vi "HLA Custom Device.Async.vi"(10 "Parameters":variant, 11 "Process":refnum<class "Process.lvclass">) -> ()   [LabVIEW 2019, in "HLA Custom Device Engine.lvlib"]
uses:
  HLA Custom Device Engine.lvlib
  <vilib>/NI/NIVS Inline Async API/_VS Inline Async API/Process/Process.lvclass
  _typedefs/AsyncDataSpace.ctl
  <vilib>/NI/NIVS Inline Async API/_Data Access Engine/Data Access Engine/Types/Write.DVR.ctl
  <vilib>/NI/NIVS Inline Async API/_Data Access Engine/Access Type Classes/Write/Write.lvclass
  <vilib>/NI/NIVS Inline Async API/_VS Inline Async API/Process/Process.lvclass/Process.ctl
  RTruntimeData.ctl
  _typedefs/RThlaMapHelpers.ctl
  _typedefs/map_in_interaction.ctl
  _typedefs/map_interaction_value.ctl
  _typedefs/map_attr_param_data.ctl
  _typedefs/map_object.ctl
  _typedefs/map_object_key.ctl
  _typedefs/map_object_value.ctl
  _typedefs/map_object_instance.ctl
  _typedefs/map_object_instance_value.ctl
  _typedefs/map_object_vs_instance.ctl
  _typedefs/map_out_vs_ch_instanceId.ctl
  _typedefs/map_out_vs_ch_objects.ctl
  _typedefs/map_out_vs_ch_objects_value.ctl
  _typedefs/map_out_vs_ch_interactIonClass.ctl
  <vilib>/addons/hla/receiveInteractionEvent_type.ctl
  <vilib>/addons/hla/OrderType.ctl
  <vilib>/addons/hla/TransportationType.ctl
  <vilib>/addons/hla/reflectAttributeValuesEvent_type.ctl
  <vilib>/addons/hla/discoverObjectInstanceEvent_type.ctl
  <vilib>/addons/hla/removeObjectInstanceEvent_type.ctl
  <vilib>/NI VeriStand/Custom Device API/Block Data Reference.ctl
  <vilib>/NI VeriStand/Custom Device API/Data Reference.ctl
  _typedefs/receiveInteraction_type.ctl
  _typedefs/interaction_info_incoming_type.ctl
  _typedefs/dataElement_type.ctl
  _typedefs/reflectAttributeValues_type.ctl
  _typedefs/object_info_received_type.ctl
  _typedefs/discoverObjectInstance_type.ctl
  <vilib>/NI/NIVS Inline Async API/_Data Access Engine/Access Type Classes/Write/Write.lvclass/Write.ctl
  <vilib>/NI/NIVS Inline Async API/_Data Access Engine/Data Access Engine/Methods/Write.Data.vi
  <vilib>/NI/NIVS Inline Async API/_VS Inline Async API/Process/Data Member Access/Read Data Access.vi
  <vilib>/NI/NIVS Inline Async API/_VS Inline Async API/Error Handling Process/SubVIs/Error.ConvertArray.vi
  <vilib>/NI/NIVS Inline Async API/_Data Access Engine/Access Type Classes/Write/Write.ProcessData.vi
  <vilib>/NI/NIVS Inline Async API/_Data Access Engine/Access Type Classes/Write/Write.Buffer.vi
  <vilib>/NI/NIVS Inline Async API/_Data Access Engine/Access Type Classes/Write/Write.Commit.vi
  Shared/Constants.vi
  <vilib>/NI/NIVS Inline Async API/_Data Access Engine/Data Access Engine/Methods/Write.Lookup.vi
  _subVIs/MessageQueue/Enqueue Message (Single).vi
  <vilib>/NI/NIVS Inline Async API/_Data Access Engine/Data Access Engine/Data Access Engine.lvclass
  Shared/HLA Custom Device Shared.lvlib
  _subVIs/MessageQueue/Message Queue.lvlib
  _subVIs/UserEvents/User Events.lvlib
  Shared/main_page_config.ctl
  Shared/object_attribute_configuration.ctl
  Shared/interaction_parameter_configuration.ctl
  Shared/Compiled.Settings.ctl
  <vilib>/addons/hla/helpers/ahvm.lvlib
  <vilib>/addons/hla/helpers/phvm.lvlib
  <vilib>/addons/hla/openrti_rti1516eLv.lvlib
  <vilib>/NI VeriStand/Custom Device API/Custom Device API.lvlib
  Shared/object_data.ctl
  Shared/object_status_info.ctl
  Shared/object_managament_config.ctl
  _Debug/VsDebugLibrary.lvlib
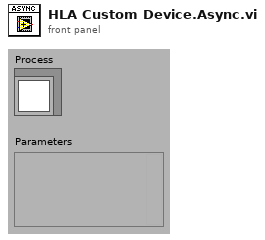
[diagram p1: front panel]
types:
  T1 = typedef "HLA Custom Device Engine.lvlib/AsyncDataSpace.ctl" = cluster{"interaction in":T2, "interaction in values":dbl[], "object in":T2, "object in values":dbl[], "status":T2, "status values":dbl[]}
  T2 = typedef "Data Access Engine.lvlib/Data Access Engine.lvclass/Write.DVR.ctl" = refnum<data-value>
  T3 = typedef "HLA Custom Device Shared.lvlib/Compiled.Settings.ctl" = cluster{"Name":string, "Async Init Timeout":u16, "main page properties":T4, "obiectConfig":T5, "objectStatus":T8, "objectData":T9}
  T4 = typedef "HLA Custom Device Shared.lvlib/main_page_config.ctl" = cluster{"Federate Execution Name":string, "Federate Type":string, "Local Designator Settings":string, "FOM Module":path, "mak mtl file":path, "FOM destination path":string, "MTL destination path":string}
  T5 = typedef "HLA Custom Device Shared.lvlib/object_managament_config.ctl" = cluster{"incoming interactions":T6[], "incoming objects":T7[], "outgoing interactions":T6[], "outgoing objects":T7[]}
  T6 = typedef "HLA Custom Device Shared.lvlib/interaction_parameter_configuration.ctl" = cluster{"interaction class name":string, "parameter name":string, "datatype":string, "vsChIndex":i32, "vsObjectId":string}
  T7 = typedef "HLA Custom Device Shared.lvlib/object_attribute_configuration.ctl" = cluster{"object class name":string, "instanceId":i32, "attribute name":string, "datatype":string, "vsChIndex":i32, "vsObjectId":string}
  T8 = typedef "HLA Custom Device Shared.lvlib/object_status_info.ctl" = cluster{"incoming interactions":map{string, map{string, i32}}, "incoming objects":map{string, map{string, i32}}, "outgoing interactions":map{string, map{string, i32}}, "outgoing objects":map{string, map{string, i32}}}
  T9 = typedef "HLA Custom Device Shared.lvlib/object_data.ctl" = cluster{"out interaction data BD":T10[], "out interaction data size":i32, "out interaction status BD":T10[], "out interaction status size":i32, "out object data BD":T10[], "out object data size":i32, "out object status BD":T10[], "out object status size":i32}
  T10 = typedef "Custom Device API.lvlib/Block Data Reference.ctl" = cluster{"Data Reference":T11, "Offset":u64, "Length":u64}
  T11 = typedef "Custom Device API.lvlib/Data Reference.ctl" = i32
  T12 = typedef "HLA Custom Device Engine.lvlib/RTruntimeData.ctl" = cluster{"rtiHandle":i64, "hlaMap":T13, "hla event registration":refnum<event-registration>, "out interaction data BD":T10[], "out interaction data":dbl[], "out interaction status BD":T10[], "out interaction status ":dbl[], "out object data BD":T10[], "out object data":dbl[], "out object status BD":T10[], "out object status ":dbl[]}
  T13 = typedef "HLA Custom Device Engine.lvlib/RThlaMapHelpers.ctl" = cluster{"in_interactionMap":T14, "in_objectMap":T17, "in_map_object_instance":T20, "in_map_vs_incoming_instance":T22, "out_map_vs_ch_instanceId":T23, "out_interactionMap":T14, "out_map_vs_ch_objectInstance":T24, "out_objectMap":T17, "out_map_vs_ch_interactionClass":T26}
  T14 = typedef "HLA Custom Device Engine.lvlib/map_in_interaction.ctl" = map{u64, T15}
  T15 = typedef "HLA Custom Device Engine.lvlib/map_interaction_value.ctl" = cluster{"infoChMap":map{string, i32}, "parameterMap":map{u64, T16}, "parHandleValueMap":u64}
  T16 = typedef "HLA Custom Device Engine.lvlib/map_attr_param_data.ctl" = cluster{"dataType":string, "offset":i32, "numOfElements":i32}
  T17 = typedef "HLA Custom Device Engine.lvlib/map_object.ctl" = map{T18, T19}
  T18 = typedef "HLA Custom Device Engine.lvlib/map_object_key.ctl" = cluster{"instanceId":i32, "objectClassHandle":u64}
  T19 = typedef "HLA Custom Device Engine.lvlib/map_object_value.ctl" = cluster{"infoChMap":map{string, i32}, "attributeMap":map{u64, T16}, "attrHandleSet":u64, "attrHandleValueMap":u64, "objectInstancePrefix":string}
  T20 = typedef "HLA Custom Device Engine.lvlib/map_object_instance.ctl" = map{u64, T21}
  T21 = typedef "HLA Custom Device Engine.lvlib/map_object_instance_value.ctl" = cluster{"objectClassHandle":u64, "objectInstanceName":string, "InstanceID":i32}
  T22 = typedef "HLA Custom Device Engine.lvlib/map_object_vs_instance.ctl" = map{u64, map{i32, u64}}
  T23 = typedef "HLA Custom Device Engine.lvlib/map_out_vs_ch_instanceId.ctl" = map{i32, i32}
  T24 = typedef "HLA Custom Device Engine.lvlib/map_out_vs_ch_objects.ctl" = map{i32, T25}
  T25 = typedef "HLA Custom Device Engine.lvlib/map_out_vs_ch_objects_value.ctl" = cluster{"objectInstanceHandle":u64, "objectClassHandle":u64}
  T26 = typedef "HLA Custom Device Engine.lvlib/map_out_vs_ch_interactIonClass.ctl" = map{i32, u64}
  T27 = typedef "HLA Custom Device Engine.lvlib/Message Queue.lvlib/All Message Queues.ctl" = cluster{"UI":refnum<queue>}
  T28 = typedef "HLA Custom Device Engine.lvlib/User Events.lvlib/userEvents_type.ctl" = cluster{"events":cluster{"stop":refnum<user-event>}, "objectNameRegNotification":refnum<notifier>}
  T29 = cluster{"Event Registration Refnum":refnum<event-registration>, "hla event registration":refnum<event-registration>}
  T30 = typedef "HLA Custom Device Engine.lvlib/receiveInteraction_type.ctl" = cluster{"interaction_info_type":T31, "dataElement[]":T34[]}
  T31 = typedef "HLA Custom Device Engine.lvlib/interaction_info_incoming_type.ctl" = cluster{"interactionHandle":u64, "Time":dbl, "TransportType":T32, "OrderType":T33}
  T32 = typedef "openrti_rti1516eLv.lvlib/TransportationType.ctl" = enum32{"null", "RELIABLE", "BEST_EFFORT"}
  T33 = typedef "openrti_rti1516eLv.lvlib/OrderType.ctl" = enum32{"null", "RECEIVE", "TIMESTAMP"}
  T34 = typedef "HLA Custom Device Engine.lvlib/dataElement_type.ctl" = cluster{"handle":u64, "dataRef":refnum<data-value>}
  T35 = typedef "HLA Custom Device Engine.lvlib/reflectAttributeValues_type.ctl" = cluster{"object_info_type":T36, "dataElement[]":T34[]}
  T36 = typedef "HLA Custom Device Engine.lvlib/object_info_received_type.ctl" = cluster{"objectInstanceHandle":u64, "Time":dbl, "TransportType":T32, "OrderType":T33}
  T37 = typedef "HLA Custom Device Engine.lvlib/discoverObjectInstance_type.ctl" = cluster{"objectInstanceHandle":u64, "objectClassHandle":u64, "objectInstanceName":string}
  T38 = cluster{"[0]":u8, "[1]":u8, "[2]":u8, "[3]":u8, "[4]":u8, "[5]":u8, "[6]":u8, "[7]":u8, "[8]":u8, "[9]":u8, "[10]":u8, "[11]":u8, "[12]":u8, "[13]":u8, "[14]":u8, "[15]":u8, "[16]":u8, "[17]":u8, "[18]":u8, "[19]":u8, "[20]":u8, "[21]":u8, "[22]":u8, "[23]":u8, "[24]":u8, "[25]":u8, "[26]":u8, "[27]":u8, "[28]":u8, "[29]":u8, "[30]":u8, "[31]":u8, "[32]":u8, "[33]":u8, "[34]":u8, "[35]":u8, "[36]":u8, "[37]":u8, "[38]":u8, "[39]":u8, "[40]":u8, "[41]":u8, "[42]":u8, "[43]":u8, "[44]":u8, "[45]":u8, "[46]":u8, "[47]":u8, "[48]":u8, "[49]":u8, "[50]":u8, "[51]":u8, "[52]":u8, "[53]":u8, "[54]":u8, "[55]":u8, "[56]":u8, "[57]":u8, "[58]":u8, "[59]":u8, "[60]":u8, "[61]":u8, "[62]":u8, "[63]":u8, "[64]":u8, "[65]":u8, "[66]":u8, "[67]":u8, "[68]":u8, "[69]":u8, "[70]":u8, "[71]":u8, "[72]":u8, "[73]":u8, "[74]":u8, "[75]":u8, "[76]":u8, "[77]":u8, "[78]":u8, "[79]":u8, "[80]":u8, "[81]":u8, "[82]":u8, "[83]":u8, "[84]":u8, "[85]":u8, "[86]":u8, "[87]":u8, "[88]":u8, "[89]":u8, "[90]":u8, "[91]":u8, "[92]":u8, "[93]":u8, "[94]":u8, "[95]":u8, "[96]":u8, "[97]":u8, "[98]":u8, "[99]":u8, "[100]":u8, "[101]":u8, "[102]":u8, "[103]":u8, "[104]":u8, "[105]":u8, "[106]":u8, "[107]":u8, "[108]":u8, "[109]":u8, "[110]":u8, "[111]":u8, "[112]":u8, "[113]":u8, "[114]":u8, "[115]":u8, "[116]":u8, "[117]":u8, "[118]":u8, "[119]":u8, "[120]":u8, "[121]":u8, "[122]":u8, "[123]":u8, "[124]":u8, "[125]":u8, "[126]":u8, "[127]":u8}
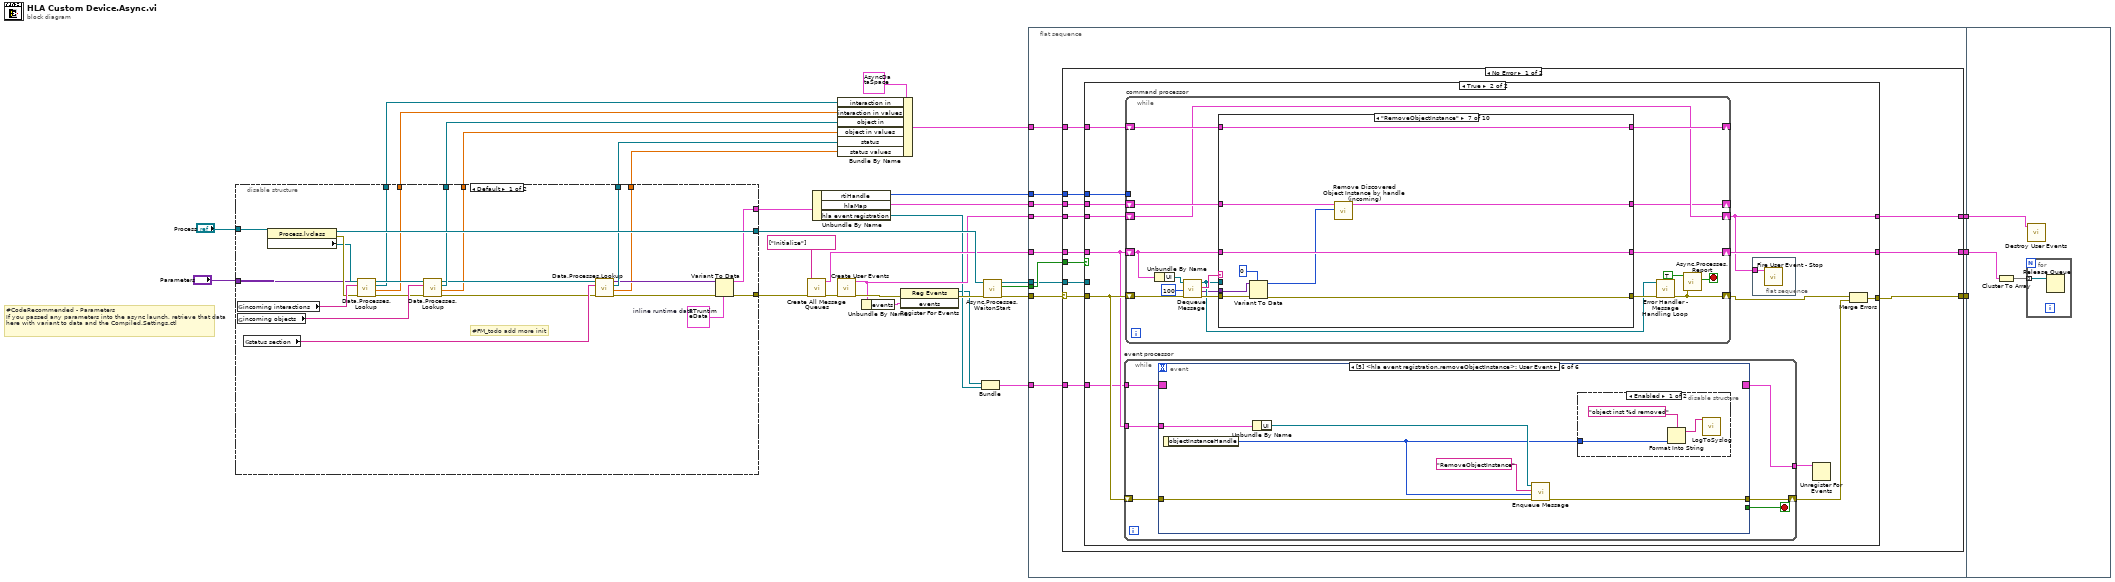
[diagram p0: block diagram]
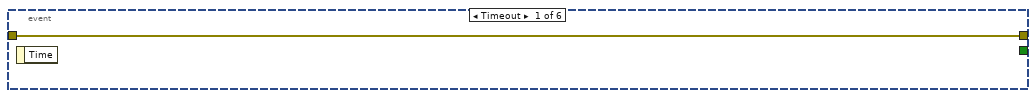
[diagram p3: hidden frame]
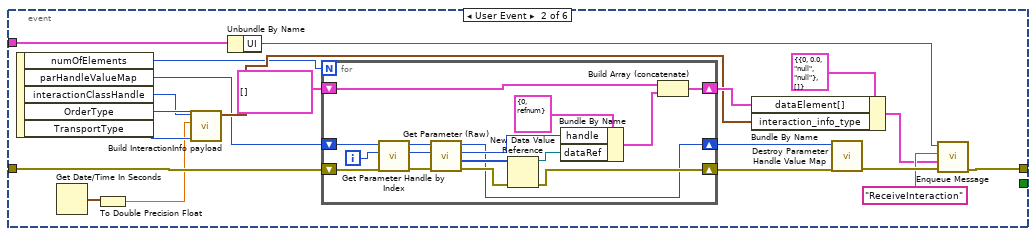
[diagram p4: hidden frame]
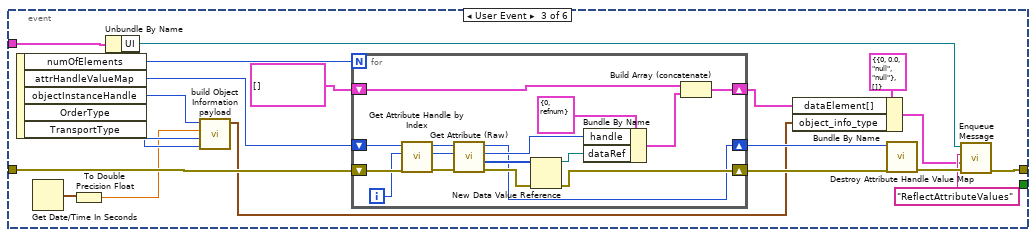
[diagram p5: hidden frame]
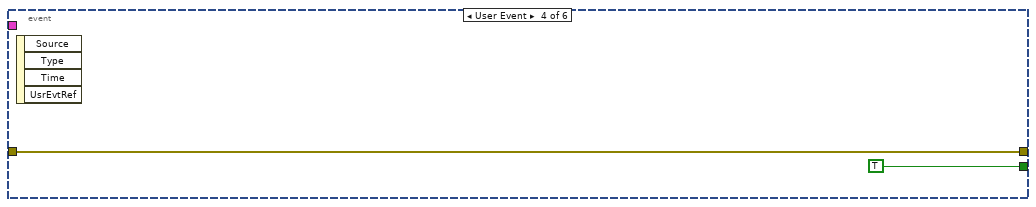
[diagram p6: hidden frame]
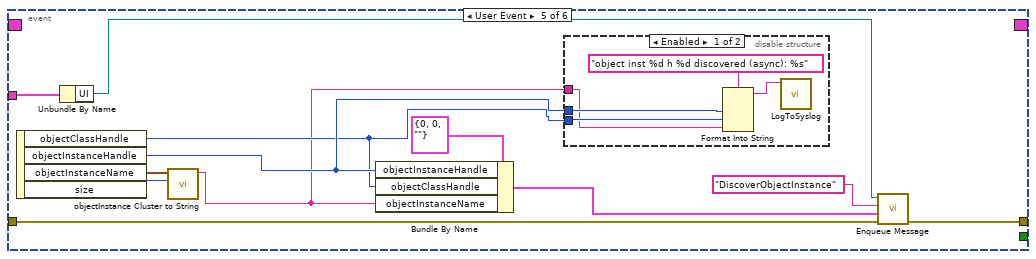
[diagram p7: hidden frame]
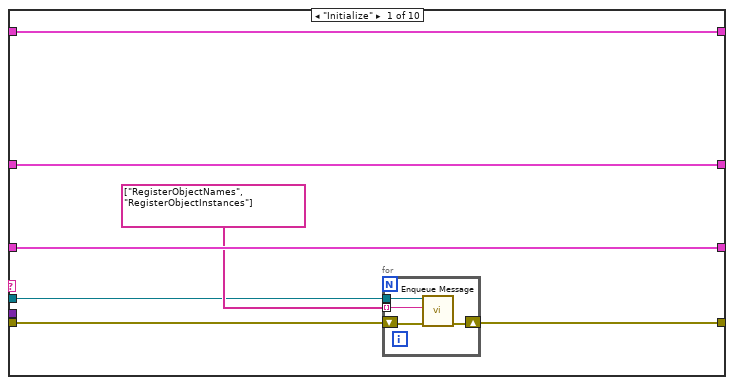
[diagram p10: hidden frame]
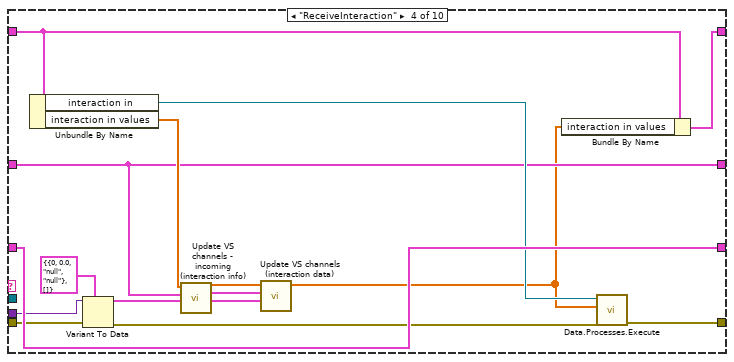
[diagram p13: hidden frame]
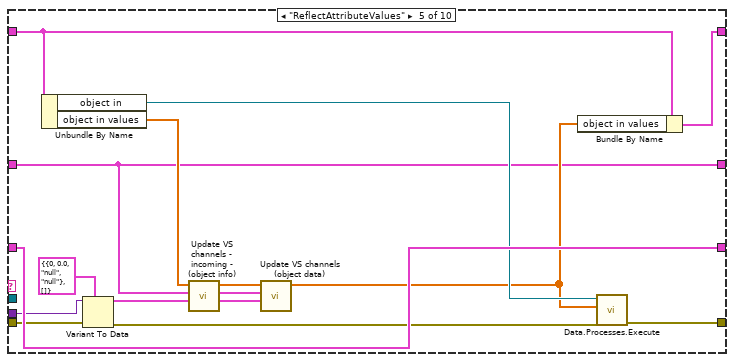
[diagram p14: hidden frame]
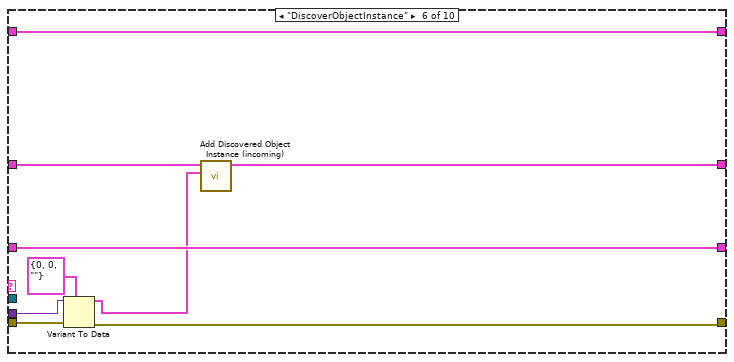
[diagram p15: hidden frame]
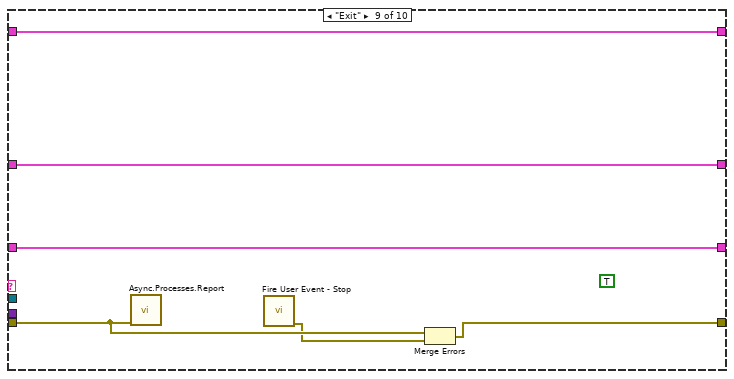
[diagram p17: hidden frame]
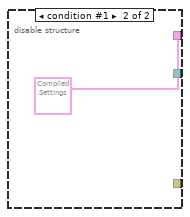
[diagram p20: hidden frame]
diagram:
  # "#CodeRecommended - Parameters\nIf you passed any parameters into the async launch, retrieve that data here with variant to data and the Compiled.Settings.ctl"
  n1 = disable-structure shown="Default" {
    disable-tunnel: "Process" -> [w47 _]
    disable-tunnel: [w46 _] -> w15
    disable-tunnel: [w45 _] -> w28
    disable-tunnel: [w44 _] -> w26
    disable-tunnel: [w41 _] -> w24
    disable-tunnel: "Parameters" -> [w37 _]
    disable-tunnel: [w36 T3 {"Name"="", "Async Init Timeout"=0, "main page properties"={"Federate Execution Name"="", "Federate Type"="", "Local Designator Settings"="", "FOM Module"=path "", "mak mtl file"=path "", "FOM destination path"="", "MTL destination path"=""}, "obiectConfig"={"incoming interactions"=[], "incoming objects"=[], "outgoing interactions"=[], "outgoing objects"=[]}, "objectStatus"={"incoming interactions"={}, "incoming objects"={}, "outgoing interactions"={}, "outgoing objects"={}}, "objectData"={"out interaction data BD"=[], "out interaction data size"=0, "out interaction status BD"=[], "out interaction status size"=0, "out object data BD"=[], "out object data size"=0, "out object status BD"=[], "out object status size"=0}} ("data")] -> w12
    disable-tunnel: [w35 w54] -> w19
    disable-tunnel: [w34 _] -> w27
    disable-tunnel: [w33 _] -> w25
    disable-tunnel: [w32 _] -> w23
    frame condition #0 (active) {
      w38 = T12 {"rtiHandle"=0, "hlaMap"={"in_interactionMap"={}, "in_objectMap"={}, "in_map_object_instance"={}, "in_map_vs_incoming_instance"={}, "out_map_vs_ch_instanceId"={}, "out_interactionMap"={}, "out_map_vs_ch_objectInstance"={}, "out_objectMap"={}, "out_map_vs_ch_interactionClass"={}}, "hla event registration"=refnum, "out interaction data BD"=[], "out interaction data"=[], "out interaction status BD"=[], "out interaction status "=[], "out object data BD"=[], "out object data"=[], "out object status BD"=[], "out object status "=[]}  # inline runtime data
      # "#FM_todo add more init"
      n2 = global read "Constants.vi" "incoming interactions"() -> (w52:string)
      n3 = global read "Constants.vi" "incoming objects"() -> (w53:string)
      n4 = global read "Constants.vi" "status section"() -> (w43:string)
      n5 = property class="Process.lvclass"(reference=w47) -> (reference out=w46:refnum<class "Process.lvclass">, error out=w51:errorcluster, "Data Member Access:Data Access"=w50:refnum<class "Data Access Engine.lvclass">)  [unwired: 1 in]
      n6 = call-poly <vilib>:"Data.Processes.Lookup.vi"("error in (no error)"=w51, "Name"=w52, "Data Access API in"=w50) -> ("error out"=w48:errorcluster, "Initial Values"=w34:dbl[], "Ref"=w45:T2, "Data Access API out"=w49:refnum<class "Data Access Engine.lvclass">)  [unwired: 5 in]
      n7 = call-poly <vilib>:"Data.Processes.Lookup.vi"("error in (no error)"=w48, "Name"=w53, "Data Access API in"=w49) -> ("error out"=w42:errorcluster, "Initial Values"=w33:dbl[], "Ref"=w44:T2, "Data Access API out"=w40:refnum<class "Data Access Engine.lvclass">)  [unwired: 5 in]
      n8 = call-poly <vilib>:"Data.Processes.Lookup.vi"("error in (no error)"=w42, "Name"=w43, "Data Access API in"=w40) -> ("error out"=w39:errorcluster, "Initial Values"=w32:dbl[], "Ref"=w41:T2)  [unwired: 5 in, 1 out]
      n9 = Variant To Data(error in=w39, type=w38, Variant=w37) -> (data=w36:T12, error out=w35:errorcluster)
    }
    frame condition #1 {
    }
  }
  n10 = call "Create All Message Queues.vi"("error in (no error)"=w19, "initialization messages"=string[] ["Initialize"]) -> ("error out"=w20:errorcluster, "Message Queues out"=w13:T27)  [unwired: 8 in]
  n11 = Unbundle By Name(w12) -> ("rtiHandle"=w11:i64, "hlaMap"=w10:T13, "hla event registration"=w6:refnum<event-registration>)
  n12 = Bundle By Name(cluster=T1 {"interaction in"=refnum, "interaction in values"=[], "object in"=refnum, "object in values"=[], "status"=refnum, "status values"=[]}, "interaction in"=w28, "interaction in values"=w27, "object in"=w26, "object in values"=w25, "status"=w24, "status values"=w23) -> (w22:T1)
  n13 = call "Create User Events.vi"("error in (no error)"=w20) -> ("error out"=w9:errorcluster, "userEvents"=w7:T28)  [unwired: 9 in]
  n14 = Unbundle By Name(w7) -> ("events"=w4:cluster{"stop":refnum<user-event>})
  n15 = register-events(error in=w9, w4) -> (reference out=w5:refnum<event-registration>, error out=w8:errorcluster)  [unwired: 1 in]
  n16 = Bundle("Event Registration Refnum"=w5, "hla event registration"=w6) -> (w3:T29)  [unwired: 1 in]
  n17 = call <vilib>:"Async.Processes.WaitonStart.vi"("error in (no error)"=w8, "Process"=w15) -> ("error out"=w18:errorcluster, "Execute"=w17:bool, "Process out"=w16:refnum<class "Process.lvclass">)  [unwired: 7 in]
  n18 = flat-sequence {
    tunnel: w22 -> [w67]
    tunnel: w18 -> [w66]
    tunnel: w17 -> [w65]
    tunnel: w16 -> [w64]
    tunnel: [w63] -> w14
    tunnel: w13 -> [w62]
    tunnel: w11 -> [w61]
    tunnel: w10 -> [w60]
    tunnel: w7 -> [w58]
    tunnel: w3 -> [w59]
    tunnel: [w57] -> w2
    tunnel: [w56] -> w1
    tunnel: w14 -> [_]
    tunnel: w2 -> [w309]
    tunnel: w1 -> [w308]
    frame #0 {
      n19 = case shown="No Error" w66 {
        selector: w66 -> [w76 w307]
        tunnel: w67 -> [w79 _]
        tunnel: w65 -> [w78 _]
        tunnel: w64 -> [w77 _]
        tunnel: [w75 w307] -> w63
        tunnel: w62 -> [w74 w306]
        tunnel: w61 -> [w73 _]
        tunnel: w60 -> [w72 _]
        tunnel: w58 -> [w71 w305]
        tunnel: w59 -> [w70 _]
        tunnel: [w69 w306] -> w57
        tunnel: [w68 w305] -> w56
        frame No Error {
          n20 = case shown="True" w78 {
            tunnel: w79 -> [_ w95]
            tunnel: w77 -> [_ _]
            tunnel: w76 -> [w82 w93]
            tunnel: [w82 w92] -> w75
            tunnel: w74 -> [w81 w91]
            tunnel: w73 -> [_ w90]
            tunnel: w72 -> [_ w89]
            tunnel: w71 -> [w80 w88]
            tunnel: w70 -> [_ w87]
            tunnel: [w81 w85] -> w69
            tunnel: [w80 w83] -> w68
            frame False {
            }
            frame True {
              n21 = while "event processor" {
                tunnel: [w102] -> w86
                shift-right: [w100] -> w94
                shift-left: w93 -> [w101]
                tunnel: w91 -> [w98]
                tunnel: w87 -> [w97]
                stop <- w99 stop-if-true
                n22 = event shown="[5] <hla event registration.removeObjectInstance>: User Event" {
                  selector: w97 -> [_ _ _ _ _ _]
                  dyn-events: [_ _ _ _ _ _] -> w102
                  timeout: _ -> [_ _ _ _ _ _]
                  tunnel: w101 -> [w103 w114 w159 w176 w181 w197]
                  tunnel: [w103 w106 w153 w176 w187 w196] -> w100
                  tunnel: [_ _ _ TRUE _ _] -> w99
                  tunnel: w98 -> [_ w109 w144 _ w185 w199]
                  event Timeout {
                    n23 = event-data() -> ()  [unwired: 1 in, 1 out]
                  }
                  event User Event {
                    n24 = event-data() -> ("numOfElements"=w111:u64, "parHandleValueMap"=w110:u64, "interactionClassHandle"=w107:u64, "OrderType"=w123:T33, "TransportType"=w122:T32)  [unwired: 1 in]
                    n25 = Get Date/Time In Seconds() -> (seconds since 1Jan1904=w105:timestamp)
                    n26 = To Double Precision Float(number=w105) -> (double precision float=w104:dbl)
                    n27 = call "Build InteractionInfo payload.vi"("TransportType"=w122, "OrderType"=w123, "Time"=w104, "interactionClassHandle"=w107) -> ("interaction_attribute_type"=w112:T31)  [unwired: 7 in]
                    n28 = Unbundle By Name(w109) -> ("UI"=w108:refnum<queue>)
                    n29 = for {
                      N: w111 -> [_]
                      shift-right: [w129] -> w120
                      shift-left: w114 -> [w139]
                      shift-right: [w124] -> w121
                      shift-left: w110 -> [w138]
                      shift-right: [w131] -> w116
                      shift-left: T34[] [] -> [w132]
                      i -> [w137]
                      n30 = call <vilib>:"Get Parameter Handle by Index.vi"("error in"=w139, "index"=w137, "parHandleValueMap in"=w138) -> ("error out"=w136:errorcluster, "parameterHandle"=w134:u64, "parHandleValueMap out"=w135:u64)  [unwired: 6 in]
                      n31 = call <vilib>:"Get Parameter (Raw).vi"("error in"=w136, "parameterHandle in"=w134, "parHandleValueMap in"=w135) -> ("error out"=w130:errorcluster, "data"=w133:u8[], "parameterHandle out"=w127:u64, "parHandleValueMap out"=w124:u64)  [unwired: 5 in]
                      n32 = New Data Value Reference(data value=w133, error in=w130) -> (data value reference=w126:refnum<data-value>, error out=w129:errorcluster)
                      n33 = Bundle By Name(cluster=T34 {"handle"=0, "dataRef"=refnum} ("dataElement"), "handle"=w127, "dataRef"=w126) -> (w125:T34)
                      n34 = Build Array (concatenate)(w132, w125) -> (w131:T34[])
                    }
                    n35 = Bundle By Name(cluster=T30 {"interaction_info_type"={"interactionHandle"=0, "Time"=0.0, "TransportType"=enum."null", "OrderType"=enum."null"}, "dataElement[]"=[]} ("receiveInteraction_type"), "dataElement[]"=w116, "interaction_info_type"=w112) -> (w115:T30)
                    n36 = call <vilib>:"Destroy Parameter Handle Value Map.vi"("error in"=w120, "attrHandleValueMap in"=w121) -> ("error out"=w119:errorcluster)  [unwired: 8 in, 1 out]
                    n37 = call-poly "Enqueue Message.vi"("error in (no error)"=w119, "Message Data"=w115, "Message"="ReceiveInteraction", "Message Queue"=w108) -> ("error out"=w106:errorcluster)  [unwired: 6 in, 1 out]
                  }
                  event User Event {
                    n38 = event-data() -> ("numOfElements"=w158:u64, "attrHandleValueMap"=w152:u64, "objectInstanceHandle"=w142:u64, "OrderType"=w151:T33, "TransportType"=w150:T32)  [unwired: 1 in]
                    n39 = Get Date/Time In Seconds() -> (seconds since 1Jan1904=w141:timestamp)
                    n40 = To Double Precision Float(number=w141) -> (double precision float=w140:dbl)
                    n41 = Unbundle By Name(w144) -> ("UI"=w143:refnum<queue>)
                    n42 = call "build Object Information payload.vi"("TransportType"=w150, "OrderType"=w151, "Time"=w140, "objectInstanceHandle"=w142) -> ("interaction_attribute_type"=w147:T36)  [unwired: 7 in]
                    n43 = for {
                      N: w158 -> [_]
                      shift-right: [w165] -> w156
                      shift-left: w159 -> [w175]
                      shift-right: [w160] -> w157
                      shift-left: w152 -> [w174]
                      shift-right: [w167] -> w146
                      shift-left: T34[] [] -> [w168]
                      i -> [w173]
                      n44 = call <vilib>:"Get Attribute Handle by Index.vi"("error in"=w175, "index"=w173, "attrHandleValueMap in"=w174) -> ("error out"=w172:errorcluster, "attributeHandle"=w170:u64, "attrHandleValueMap out"=w171:u64)  [unwired: 6 in]
                      n45 = call <vilib>:"Get Attribute (Raw).vi"("error in"=w172, "attributeHandle in"=w170, "attrHandleValueMap in"=w171) -> ("error out"=w166:errorcluster, "data"=w169:u8[], "attributeHandle out"=w163:u64, "attrHandleValueMap out"=w160:u64)  [unwired: 5 in]
                      n46 = New Data Value Reference(data value=w169, error in=w166) -> (data value reference=w162:refnum<data-value>, error out=w165:errorcluster)
                      n47 = Bundle By Name(cluster=T34 {"handle"=0, "dataRef"=refnum} ("dataElement"), "handle"=w163, "dataRef"=w162) -> (w161:T34)
                      n48 = Build Array (concatenate)(w168, w161) -> (w167:T34[])
                    }
                    n49 = Bundle By Name(cluster=T35 {"object_info_type"={"objectInstanceHandle"=0, "Time"=0.0, "TransportType"=enum."null", "OrderType"=enum."null"}, "dataElement[]"=[]} ("reflectAttributeValues_type"), "dataElement[]"=w146, "object_info_type"=w147) -> (w145:T35)
                    n50 = call <vilib>:"Destroy Attribute Handle Value Map.vi"("error in"=w156, "attrHandleValueMap in"=w157) -> ("error out"=w155:errorcluster)  [unwired: 8 in, 1 out]
                    n51 = call-poly "Enqueue Message.vi"("error in (no error)"=w155, "Message Data"=w145, "Message"="ReflectAttributeValues", "Message Queue"=w143) -> ("error out"=w153:errorcluster)  [unwired: 6 in, 1 out]
                  }
                  event User Event {
                    n52 = event-data() -> ()  [unwired: 1 in, 4 out]
                  }
                  event User Event {
                    n53 = event-data() -> ("objectClassHandle"=w179:u64, "objectInstanceHandle"=w180:u64, "objectInstanceName"=w189:T38, "size"=w188:u32)  [unwired: 1 in]
                    n54 = Unbundle By Name(w185) -> ("UI"=w184:refnum<queue>)
                    n55 = call <vilib>:"objectInstance Cluster to String.vi"("size"=w188, "string cluster in"=w189) -> ("string out"=w178:string)  [unwired: 9 in]
                    n56 = Bundle By Name(cluster=T37 {"objectInstanceHandle"=0, "objectClassHandle"=0, "objectInstanceName"=""} ("discoverObjInstance_type"), "objectInstanceHandle"=w180, "objectClassHandle"=w179, "objectInstanceName"=w178) -> (w182:T37)
                    n57 = disable-structure shown="Enabled" {
                      disable-tunnel: w180 -> [w192 _]
                      disable-tunnel: w179 -> [w191 _]
                      disable-tunnel: w178 -> [w190 _]
                      frame Enabled {
                        n58 = Format Into String(format string="object inst %d h %d discovered (async): %s", w192, w191, w190) -> (resulting string=w193:string)  [unwired: 2 in, 1 out]
                        n59 = call "LogToSyslog.vi"("message"=w193) -> ()  [unwired: 9 in, 2 out]
                      }
                      frame Disabled {
                      }
                    }
                    n60 = call-poly "Enqueue Message.vi"("error in (no error)"=w181, "Message Data"=w182, "Message"="DiscoverObjectInstance", "Message Queue"=w184) -> ("error out"=w187:errorcluster)  [unwired: 6 in, 1 out]
                  }
                  event User Event {
                    n61 = event-data() -> ("objectInstanceHandle"=w195:u64)  [unwired: 1 in]
                    n62 = Unbundle By Name(w199) -> ("UI"=w198:refnum<queue>)
                    n63 = call-poly "Enqueue Message.vi"("error in (no error)"=w197, "Message Data"=w195, "Message"="RemoveObjectInstance", "Message Queue"=w198) -> ("error out"=w196:errorcluster)  [unwired: 6 in, 1 out]
                    n64 = disable-structure shown="Enabled" {
                      disable-tunnel: w195 -> [w201 _]
                      frame Enabled {
                        n65 = Format Into String(format string="object inst %d removed", w201) -> (resulting string=w202:string)  [unwired: 2 in, 1 out]
                        n66 = call "LogToSyslog.vi"("message"=w202) -> ()  [unwired: 9 in, 2 out]
                      }
                      frame Disabled {
                      }
                    }
                  }
                }
              }
              n67 = while "command processor" {
                shift-right: [w204] -> _
                shift-left: w89 -> [w217]
                shift-right: [w218] -> w85
                shift-left: w91 -> [w207]
                shift-right: [w210] -> w84
                shift-left: w93 -> [w221]
                shift-right: [w211] -> _
                shift-left: w95 -> [w212]
                tunnel: w90 -> [_]
                shift-right: [w205] -> w83
                shift-left: w88 -> [w205]
                stop <- w209 stop-if-true
                n68 = Unbundle By Name(w207) -> ("UI"=w206:refnum<queue>)
                n69 = call "Dequeue Message.vi"("error in (no error)"=w221, "timeout in ms (-1)"=100, "Message Queue"=w206) -> ("error out"=w216:errorcluster, "Message Data"=w213:variant, "Message"=w219:string, "dup Message Queue"=w214:refnum<queue>)  [unwired: 5 in]
                n70 = case shown="\"RemoveObjectInstance\"" w219 {
                  tunnel: w207 -> [w228 w236 w240 w256 w272 w281 w290 w294 w300 w304]
                  tunnel: [w228 w236 w240 w256 w272 w281 w290 w294 w300 w304] -> w218
                  tunnel: w217 -> [w222 w233 w237 w245 w261 w276 w284 w291 w295 w301]
                  tunnel: w216 -> [w226 w235 w239 w255 w271 w279 w288 w293 w299 w303]
                  tunnel: [w224 w235 w239 w253 w269 w275 w286 w293 w297 w303] -> w215
                  tunnel: w214 -> [w225 _ _ _ _ _ _ _ _ _]
                  tunnel: w213 -> [_ _ _ w254 w270 w278 w287 _ _ _]
                  tunnel: w212 -> [w223 w234 w238 w251 w267 w280 w289 w292 w296 w302]
                  tunnel: [w223 w234 w238 w250 w266 w280 w289 w292 w296 w302] -> w211
                  tunnel: [w222 w233 w237 w245 w261 w273 w282 w291 w295 w301] -> w204
                  frame "Initialize" {
                    n71 = for {
                      tunnel: string[] ["RegisterObjectNames", "RegisterObjectInstances"] ("Message") -> [w230] mode=indexing
                      tunnel: w225 -> [w232]
                      shift-right: [w229] -> w224
                      shift-left: w226 -> [w231]
                      n72 = call-poly "Enqueue Message.vi"("error in (no error)"=w231, "Message"=w230, "Message Queue"=w232) -> ("error out"=w229:errorcluster)  [unwired: 7 in, 1 out]
                    }
                  }
                  frame "RegisterObjectNames" {
                  }
                  frame "RegisterObjectInstances" {
                  }
                  frame "ReceiveInteraction" {
                    n73 = Unbundle By Name(w251) -> ("interaction in"=w252:T2, "interaction in values"=w246:dbl[])
                    n74 = Variant To Data(error in=w255, type=T30 {"interaction_info_type"={"interactionHandle"=0, "Time"=0.0, "TransportType"=enum."null", "OrderType"=enum."null"}, "dataElement[]"=[]} ("receiveInteraction_type"), Variant=w254) -> (data=w247:T30, error out=w248:errorcluster)
                    n75 = call "Update VS channels - incoming (interaction info).vi"("receiveInteraction in"=w247, "hla map helpers in"=w245, "values in"=w246) -> ("receiveInteraction out"=w243:T30, "hla map helpers out"=w242:T13, "values out"=w244:dbl[])  [unwired: 6 in]
                    n76 = call "Update VS channels (interaction data).vi"("receiveInteraction in"=w243, "hla map helpers in"=w242, "values in"=w244) -> ("values out"=w241:dbl[])  [unwired: 6 in, 2 out]
                    n77 = Bundle By Name(cluster=w251, "interaction in values"=w241) -> (w250:T1)
                    n78 = call-poly <vilib>:"Data.Processes.Execute.vi"("error in (no error)"=w248, "Values"=w241, "Ref"=w252) -> ("error out"=w253:errorcluster)  [unwired: 8 in]
                  }
                  frame "ReflectAttributeValues" {
                    n79 = Unbundle By Name(w267) -> ("object in"=w268:T2, "object in values"=w262:dbl[])
                    n80 = Variant To Data(error in=w271, type=T35 {"object_info_type"={"objectInstanceHandle"=0, "Time"=0.0, "TransportType"=enum."null", "OrderType"=enum."null"}, "dataElement[]"=[]} ("reflectAttributeValues_type"), Variant=w270) -> (data=w259:T35, error out=w265:errorcluster)
                    n81 = call "Update VS channels - incoming - (object info).vi"("reflectAttributeValues in"=w259, "hla map helpers in"=w261, "values in"=w262) -> ("reflectAttributeValues out"=w257:T35, "hla map helpers out"=w260:T13, "values out"=w258:dbl[])  [unwired: 6 in]
                    n82 = call "Update VS channels (object data).vi"("reflectAttributeValues in"=w257, "hla map helpers in"=w260, "values in"=w258) -> ("values out"=w264:dbl[])  [unwired: 6 in, 2 out]
                    n83 = Bundle By Name(cluster=w267, "object in values"=w264) -> (w266:T1)
                    n84 = call-poly <vilib>:"Data.Processes.Execute.vi"("error in (no error)"=w265, "Values"=w264, "Ref"=w268) -> ("error out"=w269:errorcluster)  [unwired: 8 in]
                  }
                  frame "DiscoverObjectInstance" {
                    n85 = Variant To Data(error in=w279, type=T37 {"objectInstanceHandle"=0, "objectClassHandle"=0, "objectInstanceName"=""} ("discoverObjInstance_type"), Variant=w278) -> (data=w274:T37, error out=w275:errorcluster)
                    n86 = call "Add Discovered Object Instance (incoming).vi"("discoverObjInstance"=w274, "hlaMap in"=w276) -> ("hlaMap out"=w273:T13)  [unwired: 9 in]
                  }
                  frame "RemoveObjectInstance" {
                    n87 = Variant To Data(error in=w288, type=u64 0 ("objectInstanceHandle"), Variant=w287) -> (data=w283:u64, error out=w286:errorcluster)
                    n88 = call "Remove Discovered Object Instance by handle (incoming).vi"("objectInstanceHandle"=w283, "hlaMap in"=w284) -> ("hlaMap out"=w282:T13)  [unwired: 8 in, 1 out]
                  }
                  frame "Error" {
                  }
                  frame "Exit" {
                    (unwired) TRUE
                    n89 = call <vilib>:"Async.Processes.Report.vi"("Error"=w299) -> ()  [unwired: 9 in, 2 out]
                    n90 = call "Fire User Event - Stop.vi"() -> ("error out"=w298:errorcluster)  [unwired: 11 in]
                    n91 = Merge Errors(w299, w298) -> (w297:errorcluster)
                  }
                  frame "idle", Default {
                  }
                }
                n92 = call "Error Handler - Message Handling Loop.vi"("error in (no error)"=w215, "Message Queue"=w214) -> ("dup error in"=w210:errorcluster)  [unwired: 8 in, 1 out]
                n93 = call <vilib>:"Async.Processes.Report.vi"("Error"=w210, "Stop Async on Error?"=TRUE) -> ("Stop"=w209:bool)  [unwired: 8 in, 1 out]
              }
              n94 = flat-sequence {
                tunnel: w83 -> [w96]
                frame #0 {
                  n95 = call "Fire User Event - Stop.vi"("userEvents"=w96) -> ()  [unwired: 10 in, 1 out]
                }
              }
              n96 = Unregister For Events(event registration refnum=w86) -> ()  [unwired: 1 in, 1 out]
              n97 = Merge Errors(w84, w94) -> (w92:errorcluster)
            }
          }
        }
        frame Error {
        }
      }
    }
    frame #1 {
      n98 = Cluster To Array(cluster=w309) -> (array=w310:refnum<queue>[])
      n99 = for {
        tunnel: w310 -> [w311] mode=indexing
        n100 = Release Queue(queue=w311) -> ()  [unwired: 2 in, 3 out]
      }
      n101 = call "Destroy User Events.vi"("userEvents"=w308) -> ()  [unwired: 10 in, 1 out]
    }
  }
